vi "OutputAppInput.vi"(8 "error in (no error)":errorcluster, 11 "OutputToFileBasePlugin in":refnum<class "OutputToFileBasePlugin.lvclass">) -> (0 "error out":errorcluster, 2 "FilePath":path, 3 "OutputToFileBasePlugin out":refnum<class "OutputToFileBasePlugin.lvclass">)   [LabVIEW 2014, in "OutputToFilePlugins.lvlib" / "OutputToFileBasePlugin.lvclass"]
uses:
  OutputToFileBasePlugin.lvclass
  Framework/Config_class/Config.lvclass/Config.ctl
  OutputToFileBasePlugin.lvclass/OutputToFileBasePlugin.ctl
  Framework/Config_class/Accessors/Read PARTF Root Directory.vi
  Accessors/Read PmuImpairRptArray.vi
  Accessors/Read clConfigOptions.vi
  Accessors/Read OutputPath.vi
  Accessors/Read OutFileName.vi
  <vilib>/Utility/file.llb/Write To Spreadsheet File (string).vi
  Framework/Config_class/Config.lvclass
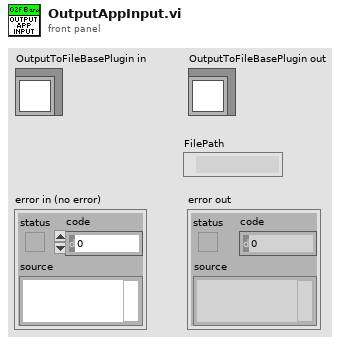
[diagram p1: front panel]
types:
  T1 = typedef "EventPlugins.lvlib/EventPluginBaseClass.lvclass/clEvtReportArray.ctl" = T2[]
  T2 = typedef "EventPlugins.lvlib/EventPluginBaseClass.lvclass/clEvtReport.ctl" = cluster{"Timestamp":dbl, "Synx":cdb[], "Freq":dbl, "ROCOF":dbl, "ID":i16}
  T3 = typedef "OutputToFilePlugins.lvlib/OutputToFileBasePlugin.lvclass/PmuCfgOpt.ctl" = cluster{"TIME_BASE":u64, "STN":string, "IDCODE":u16, "rdoPolRect":enum32{"Rectangular", "Polar"}, "rdoFloatInt":enum32{"Float", "Integer"}, "PHUNIT":u64, "rdoFreqDfreq":enum32{"Float", "Integer"}, "CHNAM":string[], "chkCfg2Prefix":bool}
  T4 = typedef "Framework.lvlib/Config.lvclass/RootDir.ctl" = cluster{"pathRootDir":path, "btnOutPath":bool, "OutDir":string, "btnOpenOutputDir":bool, "ScriptDir":string, "btnOpenScriptDir":bool, "TestDir":string, "btnOpenTestDir":bool}
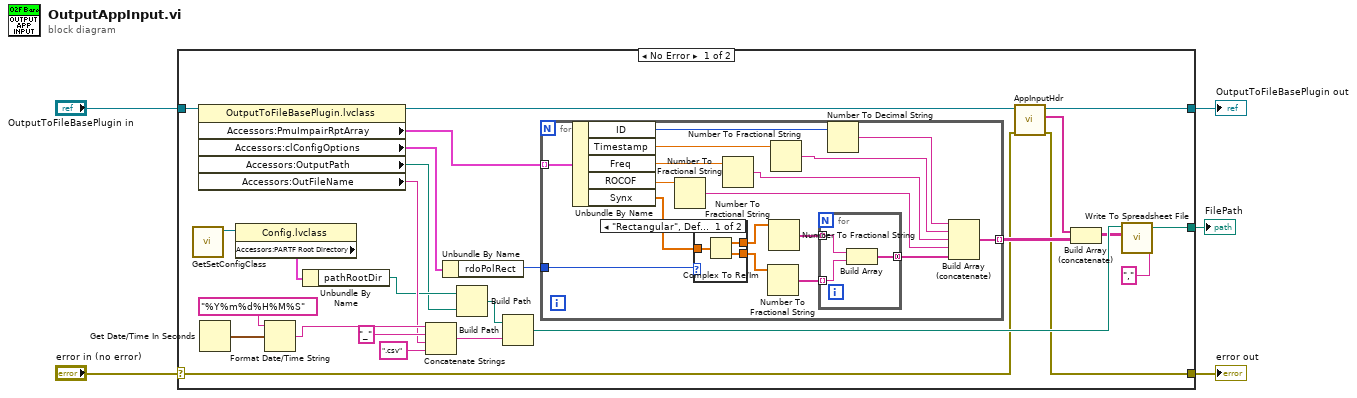
[diagram p0: block diagram]
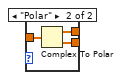
[diagram p2: hidden frame]
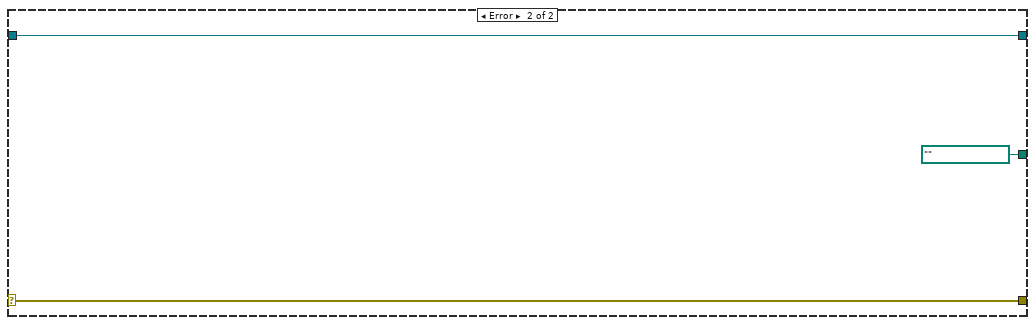
[diagram p3: hidden frame]
diagram:
  n1 = case shown="No Error" "error in (no error)" {
    selector: "error in (no error)" -> [w12 w60]
    tunnel: [w11 w60] -> w4
    tunnel: [w23 w59] -> w2
    tunnel: "OutputToFileBasePlugin in" -> [w31 w59]
    tunnel: [w13 path "" ("new file path (Not A Path if cancelled)")] -> w1
    frame No Error {
      n2 = call "GetSetConfigClass.vi"() -> ("Ref out"=w10:refnum<class "Config.lvclass">)  [unwired: 11 in]
      n3 = property class="OutputToFileBasePlugin.lvclass"(reference=w31) -> (reference out=w24:refnum<class "OutputToFileBasePlugin.lvclass">, "Accessors:PmuImpairRptArray"=w19:T1, "Accessors:clConfigOptions"=w21:T3, "Accessors:OutputPath"=w6:path, "Accessors:OutFileName"=w22:string)  [unwired: 1 in, 1 out]
      n4 = Get Date/Time In Seconds() -> (seconds since 1Jan1904=w30:timestamp)
      n5 = property class="Config.lvclass"(reference=w10) -> ("Accessors:PARTF Root Directory"=w9:T4)  [unwired: 1 in, 2 out]
      n6 = Format Date/Time String(time format string (%c)="%Y%m%d%H%M%S", seconds (now)=w30) -> (date/time string=w28:string)  [unwired: 1 in]
      n7 = Unbundle By Name(w9) -> ("pathRootDir"=w7:path)
      n8 = Concatenate Strings(w28, "_" ("string"), w22, ".csv" ("string")) -> (w25:string)
      n9 = Unbundle By Name(w21) -> ("rdoPolRect"=w20:enum32{"Rectangular", "Polar"})
      n10 = Build Path(base path=w7, name or relative path=w6) -> (appended path=w8:path)
      n11 = Build Path(base path=w8, name or relative path=w25) -> (appended path=w16:path)
      n12 = for {
        tunnel: w20 -> [w48]
        tunnel: w19 -> [w43] mode=indexing
        tunnel: [w32] -> w17 mode=indexing
        n13 = Unbundle By Name(w43) -> ("ID"=w37:i16, "Timestamp"=w38:dbl, "Freq"=w39:dbl, "ROCOF"=w40:dbl, "Synx"=w42:cdb[])
        n14 = Number To Fractional String(number=w40) -> (F-format string=w36:string)  [unwired: 3 in]
        n15 = case shown="\"Rectangular\", Default" w48 {
          tunnel: w42 -> [w54 w57]
          tunnel: [w52 w56] -> w47
          tunnel: [w53 w55] -> w46
          frame "Rectangular", Default {
            n16 = Complex To Re/Im(x + iy=w54) -> (x=w52:dbl[], y=w53:dbl[])
          }
          frame "Polar" {
            n17 = Complex To Polar(r * e^(i*theta)=w57) -> (r=w56:dbl[], theta=w55:dbl[])
          }
        }
        n18 = Number To Fractional String(number=w39) -> (F-format string=w35:string)  [unwired: 3 in]
        n19 = Number To Fractional String(number=w46) -> (F-format string=w44:string[])  [unwired: 3 in]
        n20 = Number To Fractional String(number=w47) -> (F-format string=w45:string[])  [unwired: 3 in]
        n21 = Number To Fractional String(number=w38) -> (F-format string=w34:string)  [unwired: 3 in]
        n22 = for {
          tunnel: w45 -> [w50] mode=indexing
          tunnel: w44 -> [w51] mode=indexing
          tunnel: [w49] -> w41 mode=concatenating
          n23 = Build Array(w50, w51) -> (w49:string[])
        }
        n24 = Number To Decimal String(number=w37) -> (decimal integer string=w33:string)  [unwired: 1 in]
        n25 = Build Array (concatenate)(w33, w34, w35, w36, w41) -> (w32:string[])
      }
      n26 = call "AppInputHdr.vi"("error in (no error)"=w12, "OutputToFileBasePlugin in"=w24) -> ("error out"=w11:errorcluster, "Header"=w18:string[], "OutputToFileBasePlugin out"=w23:refnum<class "OutputToFileBasePlugin.lvclass">)  [unwired: 7 in]
      n27 = Build Array (concatenate)(w18, w17) -> (w15:string[][])
      n28 = call-poly <vilib>:"Write To Spreadsheet File.vi"("delimiter (\\t)"="," ("delimiter (\\t)"), "2D data"=w15, "file path (dialog if empty)"=w16) -> ("new file path (Not A Path if cancelled)"=w13:path)  [unwired: 5 in]
    }
    frame Error {
    }
  }
  "error out" <- w4
  "OutputToFileBasePlugin out" <- w2
  "FilePath" <- w1
